vi "GetPosition.vi"(8 "error in (no error)":errorcluster, 11 "text item in":refnum<class "text item.lvclass">) -> (0 "error out":errorcluster, 2 "position":cluster{"left":u32, "top":u32}, 3 "text item out":refnum<class "text item.lvclass">)   [LabVIEW 2009, in "text item.lvclass"]
uses:
  text item.lvclass
  text item.lvclass/text item.ctl
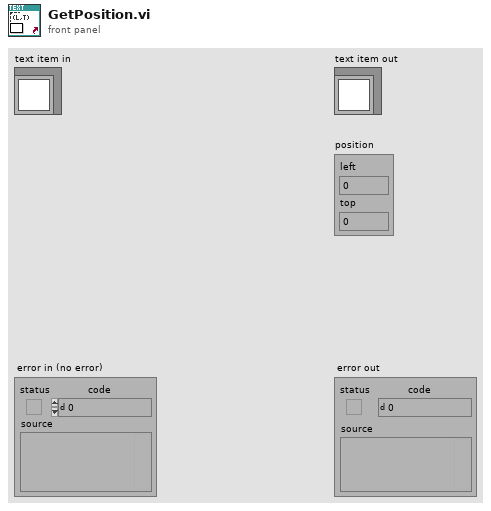
[diagram p1: front panel]
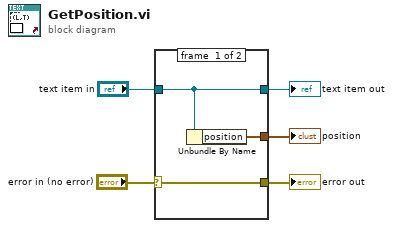
[diagram p0: block diagram]
diagram:
  n1 = case shown="No Error" "error in (no error)" {
    selector: "error in (no error)" -> [w6 w9]
    tunnel: [w8 _] -> w5
    tunnel: "text item in" -> [w7 w10]
    tunnel: [w7 w10] -> w3
    tunnel: [w6 w9] -> w1
    frame #0 {
      n2 = Unbundle By Name(w7) -> ("position"=w8:cluster{"left":u32, "top":u32})
    }
    frame #1 {
    }
  }
  "error out" <- w1
  "text item out" <- w3
  "position" <- w5
